vi "LJUD_eGetS.vi"(5 "Channel":i32, 7 "IOType":string, 8 "error in":errorcluster, 9 "x1":i32, 10 "Value Write":dbl format="%.2f", 11 "Handle In":i32) -> (0 "error out":errorcluster, 2 "Value Read":dbl format="%.2f", 3 "Handle Out":i32)   [LabVIEW 2020]
doc: "In this version of eGet the\nIOType is a string.\n\nThis is a traditional technique UD\nfunction that internally performs\na single Add, a GoOne, and a single\nGet. See Section 4.1 of the device's\ndatasheet for more information.\n\nIOType specifies what sort of action\nwill be performed. The other inputs\ndepend on the IOType. See the\npseudocode in Section 4.3 for info."
uses:
  labjackud.dll
panel:
  # "In this version of eGet the\nIOType is a string.\n\nThis is a traditional technique UD\nfunction that internally performs\na single Add, a GoOne, and a single\nGet.  See Section 4.1 of the device's\ndatasheet for more information.\n\nIOType specifies what sort of action\nwill be performed.  The other inputs\ndepend on the IOType.  See the\npseudocode in Section 4.3 for info."
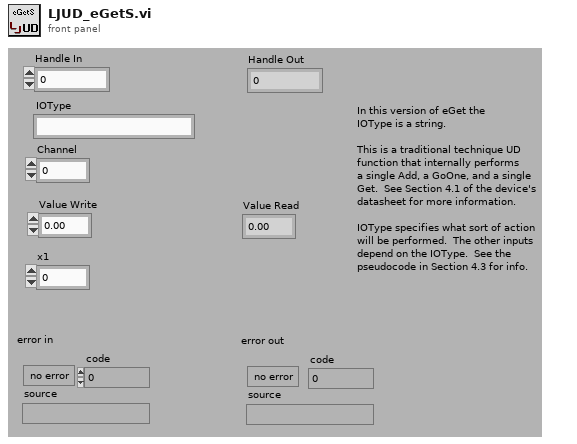
[diagram p1: front panel]
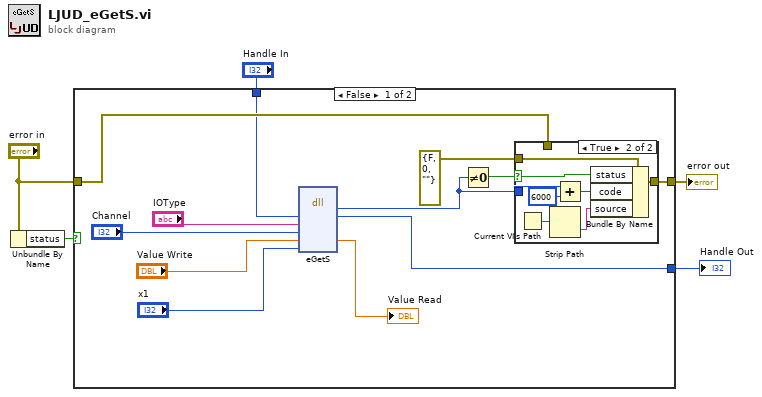
[diagram p0: block diagram]
diagram:
  n1 = Unbundle By Name("error in") -> ("status"=w4:bool)
  n2 = case shown="False" w4 {
    tunnel: [w9 w28] -> w5
    tunnel: "error in" -> [w8 w28]
    tunnel: "Handle In" -> [w7 w27]
    tunnel: [w6 w27] -> w1
    frame False {
      n3 = dll-call lib="labjackud.dll" fn="eGetS"("Handle"=w7, "IOType"="IOType", "Channel"="Channel", "Value"="Value Write", "x1"="x1") -> (w10:i32, "Handle"=w6:i32, "Value"=→"Value Read":dbl)  [unwired: 6 in, 2 out]
      n4 = Not Equal To 0?(x=w10) -> (x != 0?=w11:bool)
      n5 = case shown="True" w11 {
        selector: w11 -> [_ w25]
        tunnel: [w18 w26] -> w9
        tunnel: errorcluster {"status"=FALSE, "code"=0, "source"=""} ("error IO") -> [_ w24]
        tunnel: w10 -> [_ w20]
        tunnel: w8 -> [w18 _]
        frame False {
        }
        frame True {
          n6 = Current VI's Path() -> (path=w22:path)
          n7 = Strip Path(path=w22) -> (name=w23:string)  [unwired: 1 out]
          n8 = Add(x=w20, y=6000) -> (x+y=w21:i32)
          n9 = Bundle By Name(cluster=w24, "status"=w25, "code"=w21, "source"=w23) -> (w26:errorcluster)
        }
      }
    }
    frame True {
    }
  }
  "error out" <- w5
  "Handle Out" <- w1
